vi "AudioSetup.vi"() -> ()   [LabVIEW 2014]
uses:
  Element.ctl
  States.ctl
  <vilib>/Analysis/4window.llb/windowTd.ctl
  <vilib>/Instr/_visa.llb/VISA Configure Serial Port (Instr).vi
  <vilib>/Analysis/NI_AALPro.lvlib
  <vilib>/gmath/NI_Gmath.lvlib
panel:
  out "Elements Out":T1[](array[typedef])
  in  "stop":bool
  in  "Offset Volt":dbl
  in  "Visualizers":T2(tab)
  out "Local Signal":dbl[](graph)
  out "Global Signal":dbl[](graph)
  out "Intensity Graph":dbl[][](graph)
  out "Local Signal FFT":dbl[](graph)
  in  "Controls & Indicators":T3(tab)
  in  "Port Config Control":T4={"Baudrate"=2000000, "COM Port"="", "Termination\nCharacter"=10} {"Termination\nCharacter" format="%.0x"}
  in  "ADC Config Control":T5={"Resolution"=8, "VCC"=5.0, "Sampling Frequency"=75000.0, "Data Blocks"=20, "Samples per Block"=200} {"Data Blocks" min=1 max=50000 step=1}
  out "ADC Config Indicator":cluster{"Number of Samples":u32}
  in  "Record Config Control":T6={"index"=76000, "Freq. Res 2"=0.0, "time steps"=-1, "frequency bins"=512, "type"=enum."", "length"=64}
  in  "FFT Config Control":T7={"time steps"=-1, "frequency bins"=512, "length"=64, "Freq. Res"=0.0, "type"=enum."Rectangle"}
  out "count 2":i32
  out "Acquisition Loop":dbl format="%.4p"
  out "VISA Loop":dbl format="%.4p"
  out "FFT Loop":dbl format="%.4p"
  out "Main Loop":dbl format="%.4p"
  in  "Menu Cluster":T8
  in  "Menu Button":bool
  in  "Lock Gate":bool
  in  "Parar":bool
  in  "Gate":bool
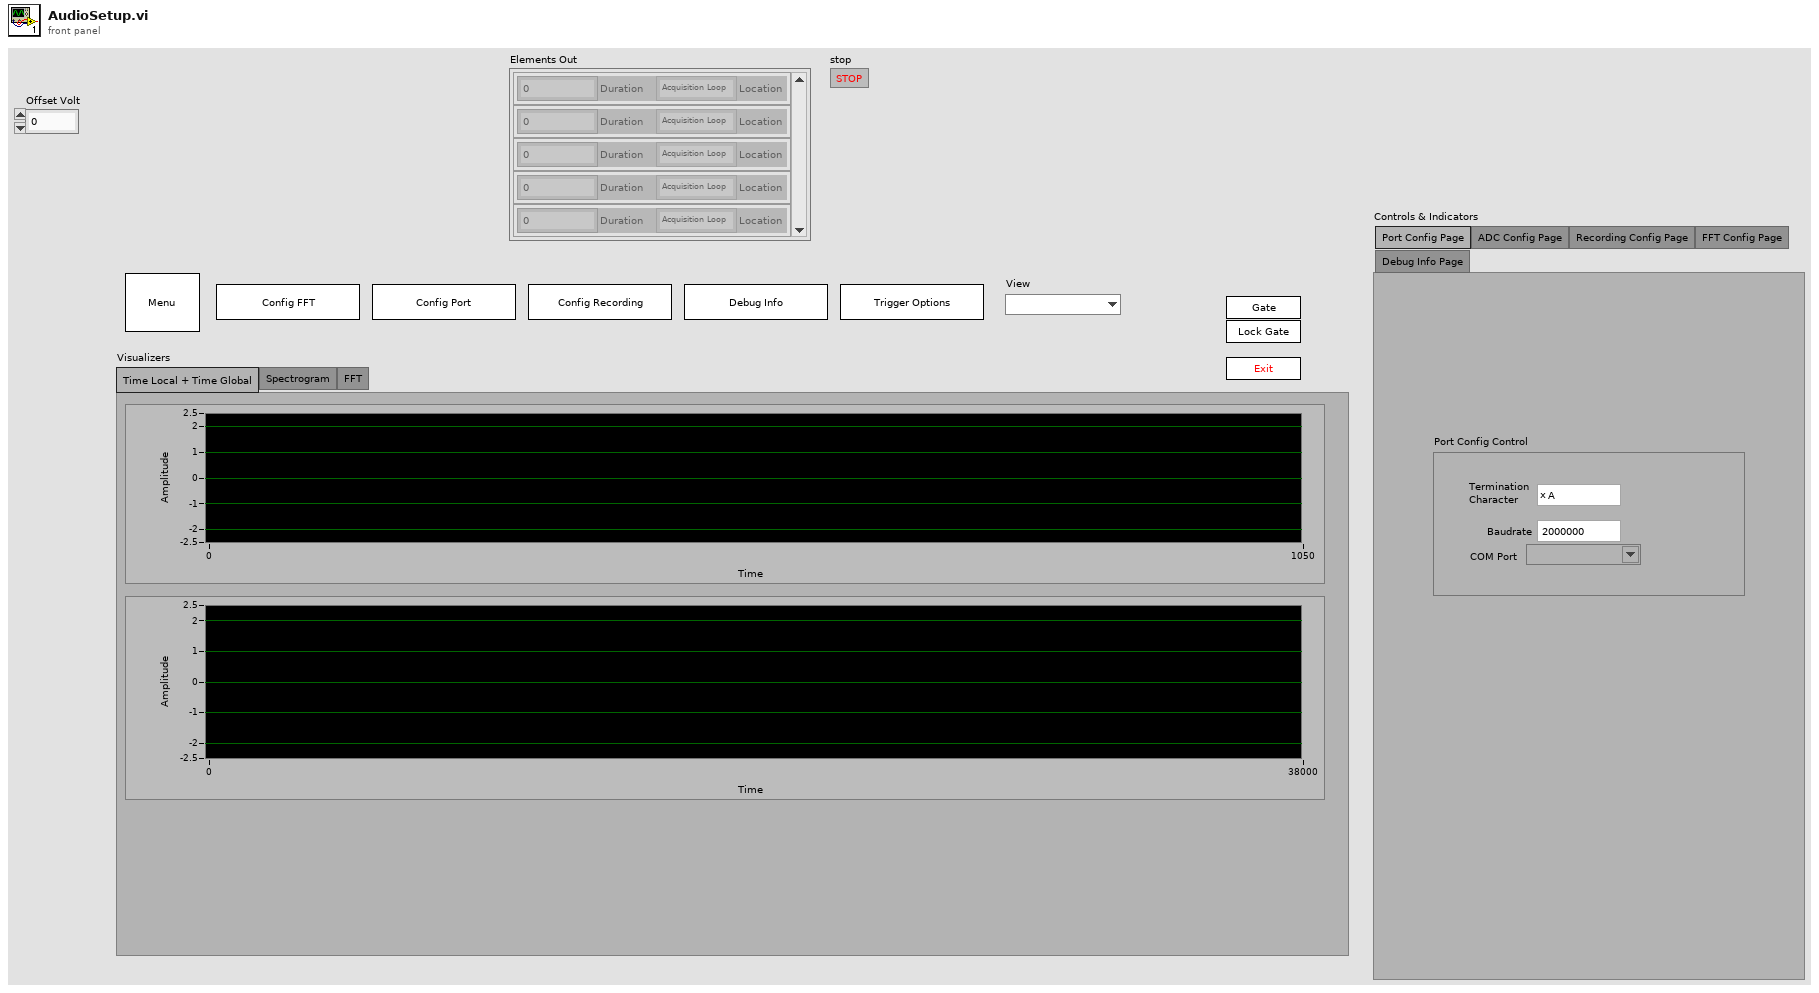
[diagram p1: front panel]
types:
  T1 = typedef "Element.ctl" = cluster{"Duration":dbl, "Location":enum16{"Acquisition Loop", "VISA Loop", "FFT Loop", "Spectrogram Loop"}}
  T2 = enum32{"Time Local + Time Global", "Spectrogram", "FFT"}
  T3 = enum32{"Port Config Page", "ADC Config Page", "Recording Config Page", "FFT Config Page", "Debug Info Page"}
  T4 = cluster{"Baudrate":u32, "COM Port":refnum<visa-resource-name>, "Termination\nCharacter":u8}
  T5 = cluster{"Resolution":i16, "VCC":dbl, "Sampling Frequency":dbl, "Data Blocks":u32, "Samples per Block":u32}
  T6 = cluster{"index":i32, "Freq. Res 2":dbl, "time steps":i32, "frequency bins":i32, "type":enum16{""}, "length":i32}
  T7 = cluster{"time steps":i32, "frequency bins":i32, "length":i32, "Freq. Res":dbl, "type":enum16{"Rectangle", "Hanning", "Hamming", "Blackman-Harris", "Exact Blackman", "Blackman", "Flat Top", "4 Term B-Harris ", "7 Term B-Harris", "Low Sidelobe", "Blackman Nuttall", "Triangle", "Bartlett-Hanning", "Bohman", "Parzen", "Welch", "Kaiser", "Dolph-Chebyshev", "Gaussian"}}
  T8 = cluster{"Configure FFT Parameters":bool, "Configure Comunication Port":bool, "Recording Options":bool, "Debug Info":bool, "Trigger Options":bool, "View":enum16{""}}
  T9 = typedef "States.ctl" = enum16{"Init", "Flush", "Add"}
  T10 = typedef "NI_AALPro.lvlib/windowTd.ctl" = enum16{"Rectangle", "Hanning", "Hamming", "Blackman-Harris", "Exact Blackman", "Blackman", "Flat Top", "4 Term B-Harris ", "7 Term B-Harris", "Low Sidelobe", "Blackman Nuttall", "Triangle", "Bartlett-Hanning", "Bohman", "Parzen", "Welch", "Kaiser", "Dolph-Chebyshev", "Gaussian"}
  T11 = enum16{"Rectangle", "Hanning", "Hamming", "Blackman-Harris", "Exact Blackman", "Blackman", "Flat Top", "4 Term B-Harris ", "7 Term B-Harris", "Low Sidelobe", "Blackman Nuttall", "Triangle", "Bartlett-Hanning", "Bohman", "Parzen", "Welch", "Kaiser", "Dolph-Chebyshev", "Gaussian"}
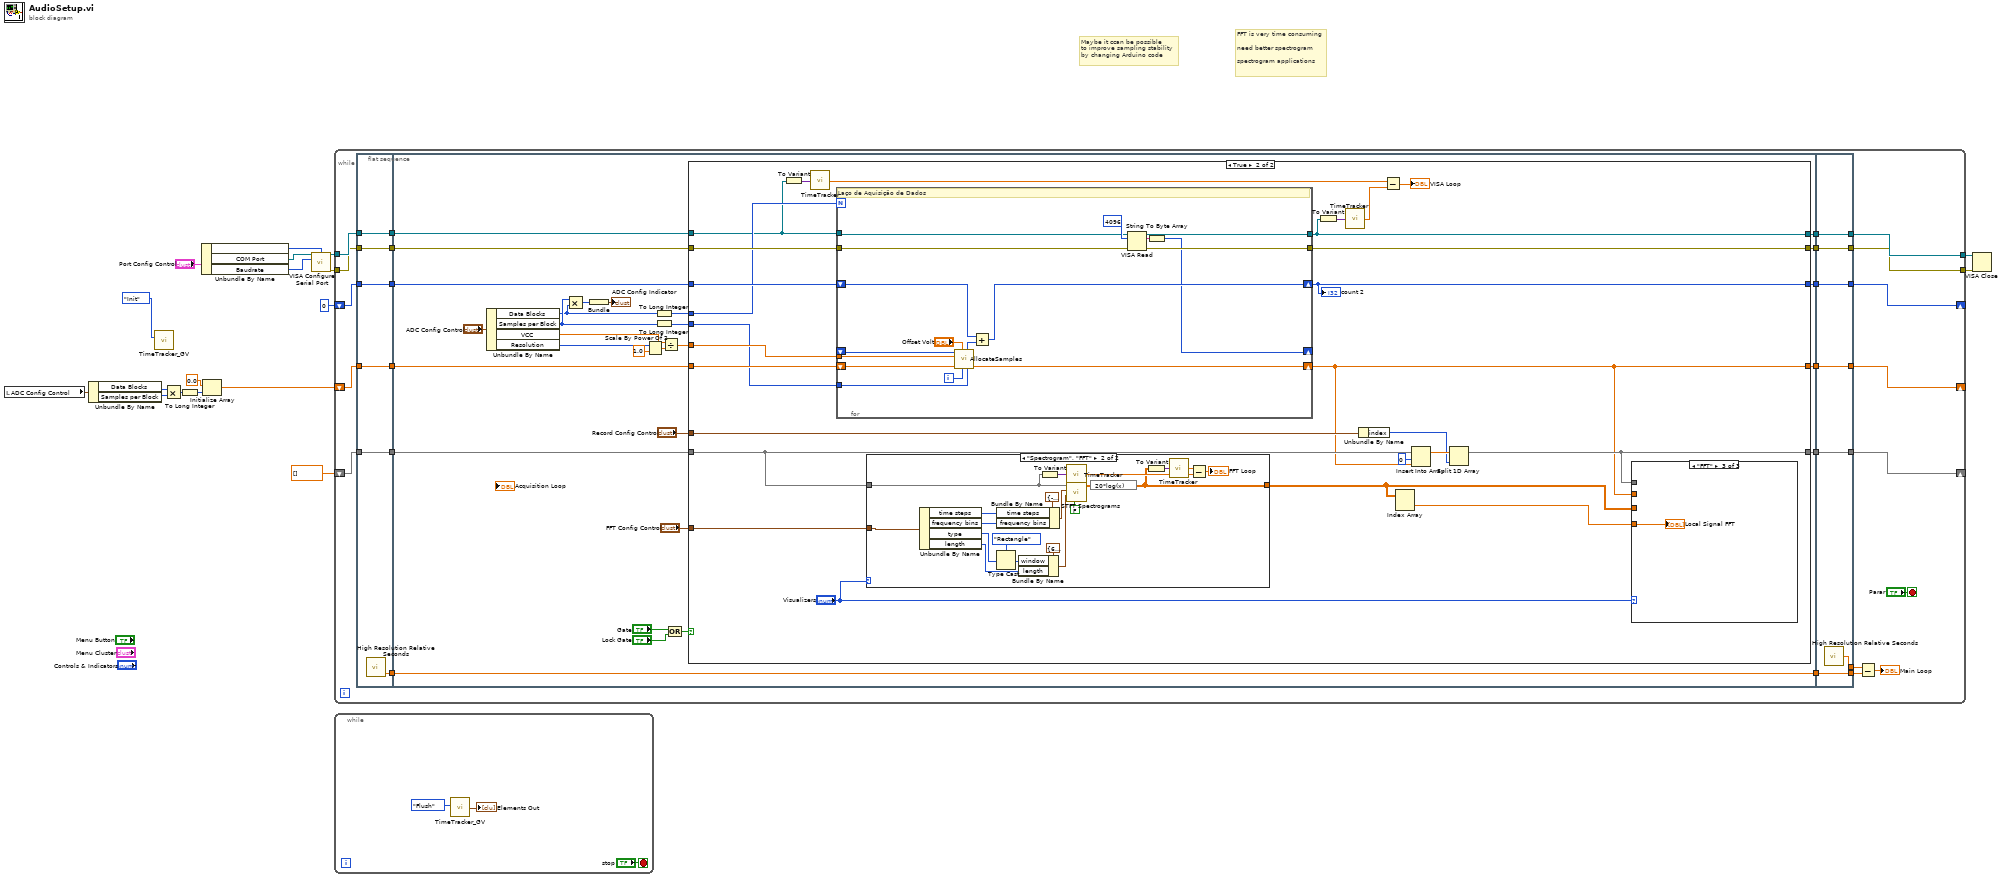
[diagram p0: block diagram]
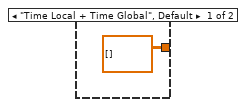
[diagram p3: hidden frame]
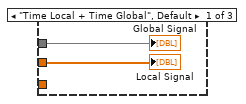
[diagram p4: hidden frame]
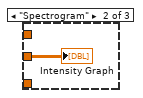
[diagram p5: hidden frame]
diagram:
  # "FFT is very time consuming\n\nneed better spectrogram\n\nspectrogram applications"
  # "Maybe it ccan be possible \nto improve sampling stability \nby changing Arduino code"
  n1 = local read "ADC Config Control"() -> (w5:T5)
  n2 = Unbundle By Name(w5) -> ("Data Blocks"=w4:u32, "Samples per Block"=w3:u32)
  n3 = call "TimeTracker_GV.vi"("Action"=States."Init") -> ()  [unwired: 6 in, 1 out]
  n4 = Multiply(x=w4, y=w3) -> (x*y=w2:u32)
  n5 = To Long Integer(number=w2) -> (32bit integer=w12:i32)
  n6 = Unbundle By Name("Port Config Control") -> ("Termination\nCharacter"=w8:u8, "COM Port"=w7:refnum<visa-resource-name>, "Baudrate"=w6:u32)
  n7 = Initialize Array(0.0 ("dimension size"), w12) -> (w13:dbl[])
  n8 = call-poly "VISA Configure Serial Port"("VISA resource name"=w7, "termination char\n(0xA = '\\n' = LF)"=w8, "baud rate (9600)"=w6) -> ("VISA resource name out"=w18:refnum<visa-resource-name>, "error out"=w17:errorcluster)  [unwired: 11 in]
  n9 = while {
    tunnel: w18 -> [w44]
    tunnel: w17 -> [w41]
    tunnel: [w43] -> w16
    tunnel: [w42] -> w15
    shift-right: [w38] -> _
    shift-left: 0 ("dimension size") -> [w39]
    shift-right: [w37] -> _
    shift-left: w13 -> [w40]
    shift-right: [w36] -> _
    shift-left: dbl[] [] -> [w35]
    stop <- "Parar" stop-if-true
    n10 = flat-sequence {
      tunnel: w35 -> [w46]
      tunnel: w39 -> [w47]
      tunnel: w40 -> [w48]
      tunnel: w41 -> [w49]
      tunnel: w44 -> [w50]
      tunnel: [w50] -> w29
      tunnel: [w49] -> w28
      tunnel: [w48] -> w27
      tunnel: [w47] -> w26
      tunnel: [w46] -> w25
      tunnel: [w45] -> w21
      tunnel: [w77] -> w34
      tunnel: [w76] -> w33
      tunnel: [w69] -> w32
      tunnel: [w68] -> w31
      tunnel: [w67] -> w30
      tunnel: w29 -> [w78]
      tunnel: w28 -> [w72]
      tunnel: w27 -> [w71]
      tunnel: w26 -> [w70]
      tunnel: w25 -> [w66]
      tunnel: w21 -> [w51]
      tunnel: [w51] -> w20
      tunnel: [w154] -> w36
      tunnel: [w155] -> w37
      tunnel: [w156] -> w38
      tunnel: [w157] -> w42
      tunnel: [w158] -> w43
      tunnel: w34 -> [w158]
      tunnel: w33 -> [w157]
      tunnel: w32 -> [w156]
      tunnel: w31 -> [w155]
      tunnel: w30 -> [w154]
      tunnel: [w153] -> w22
      tunnel: w20 -> [w152]
      tunnel: [w152] -> w19
      frame #0 {
        n11 = call <vilib>:"High Resolution Relative Seconds.vi"() -> ("relative seconds"=w45:dbl)
      }
      frame #1 {
        n12 = Unbundle By Name("ADC Config Control") -> ("Data Blocks"=w54:u32, "Samples per Block"=w55:u32, "VCC"=w62:dbl, "Resolution"=w63:i16)
        n13 = Multiply(x=w55, y=w54) -> (x*y=w52:u32)
        n14 = Bundle(w52) -> (→"ADC Config Indicator":cluster{u32})  [unwired: 1 in]
        n15 = Scale By Power Of 2(n=w63, x=1.0) -> (x*2^n=w60:dbl)
        n16 = To Long Integer(number=w54) -> (32bit integer=w56:i32)
        n17 = To Long Integer(number=w55) -> (32bit integer=w57:i32)
        n18 = Divide(x=w62, y=w60) -> (x/y=w59:dbl)
        n19 = Or(x="Gate", y="Lock Gate") -> (x .or. y?=w73:bool)
        n20 = case shown="True" w73 {
          tunnel: w78 -> [w83 w87]
          tunnel: w72 -> [w82 w108]
          tunnel: [w83 w88] -> w77
          tunnel: [w82 w109] -> w76
          tunnel: w71 -> [w80 w107]
          tunnel: w70 -> [w81 w106]
          tunnel: [w81 w105] -> w69
          tunnel: w59 -> [_ w104]
          tunnel: [w80 w99] -> w68
          tunnel: [w79 w102] -> w67
          tunnel: w66 -> [w79 w103]
          tunnel: "FFT Config Control" -> [_ w101]
          tunnel: "Record Config Control" -> [_ w100]
          tunnel: w57 -> [_ w98]
          tunnel: w56 -> [_ w97]
          frame False {
          }
          frame True {
            n21 = To Variant(anything=w87) -> (Variant=w89:variant)
            n22 = call "TimeTracker.vi"("Ref In"=w89) -> ("Time Out"=w86:dbl)  [unwired: 4 in]
            n23 = for {
              N: w97 -> [_]
              tunnel: w87 -> [w140]
              tunnel: w108 -> [w146]
              tunnel: [w141] -> w88
              tunnel: [w145] -> w109
              shift-right: [w132] -> w99
              shift-left: w107 -> [w131]
              tunnel: w98 -> [w133]
              shift-right: [w143] -> w105
              shift-left: w106 -> [w142]
              shift-right: [w139] -> _
              shift-left: _ -> [w137]
              tunnel: w104 -> [w136]
              i -> [w135]
              # "Laço de Aquisição de Dados"
              n24 = call "AllocateSamples.vi"("Samples per Block"=w133, "Loop Iteration"=w135, "Offset Volt"="Offset Volt", "Converted Array In"=w131, "Conversion Constant"=w136, "Raw Array In"=w137) -> ("Converted Array out"=w132:dbl[], "Missed Samples"=w134:i32)  [unwired: 3 in, 1 out]
              n25 = Add(x=w142, y=w134) -> (x+y=w143:i32)
              n26 = VISA Read(VISA resource name=w140, byte count=u32 4096, error in (no error)=w146) -> (VISA resource name out=w141:refnum<visa-resource-name>, read buffer=w144:string, error out=w145:errorcluster)  [unwired: 1 out]
              n27 = String To Byte Array(string=w144) -> (unsigned byte array=w139:u8[])
            }
            "count 2" <- w105
            n28 = case shown="\"Spectrogram\", \"FFT\"" "Visualizers" {
              tunnel: w101 -> [_ w117]
              tunnel: [dbl[][] [] ("STFT Spectrogram {X}") w113] -> w96
              tunnel: w103 -> [_ w111]
              frame "Time Local + Time Global", Default {
              }
              frame "Spectrogram", "FFT" {
                n29 = Unbundle By Name(w117) -> ("time steps"=w126:i32, "frequency bins"=w125:i32, "type"=w119:T11, "length"=w123:i32)
                n30 = Type Cast(type=windowTd."Rectangle", x=w119) -> (*(type *) &x=w120:T10)
                n31 = Bundle By Name(cluster=cluster{"time steps":i32, "frequency bins":i32} {"time steps"=-1, "frequency bins"=512} ("time-freq sampling info"), "time steps"=w126, "frequency bins"=w125) -> (w124:cluster{"time steps":i32, "frequency bins":i32})
                n32 = Bundle By Name(cluster=cluster{"length":i32, "window":T10} {"length"=64, "window"=enum."Rectangle"} ("window info"), "window"=w120, "length"=w123) -> (w122:cluster{"length":i32, "window":T10})
                n33 = To Variant(anything=w111) -> (Variant=w112:variant)
                n34 = call "TimeTracker.vi"("Ref In"=w112) -> ("Time Out"=w115:dbl)  [unwired: 4 in]
                n35 = call <vilib>:"STFT Spectrograms.vi"("energy conservation?"=FALSE, "window info"=w122, "time-freq sampling info"=w124, "X"=w111) -> ("STFT Spectrogram {X}"=w128:dbl[][])  [unwired: 6 in, 1 out]
                n36 = expression code="20*log(x)"(w128) -> (w113:dbl[][])
                n37 = To Variant(anything=w113) -> (Variant=w114:variant)
                n38 = call "TimeTracker.vi"("Ref In"=w114) -> ("Time Out"=w116:dbl)  [unwired: 4 in]
                n39 = Subtract(x=w116, y=w115) -> (x-y=→"FFT Loop":dbl)
              }
            }
            n40 = To Variant(anything=w88) -> (Variant=w90:variant)
            n41 = call "TimeTracker.vi"("Ref In"=w90) -> ("Time Out"=w85:dbl)  [unwired: 4 in]
            n42 = Unbundle By Name(w100) -> ("index"=w91:i32)
            n43 = Subtract(x=w86, y=w85) -> (x-y=→"VISA Loop":dbl)
            n44 = Index Array(array=w96) -> (element=w95:dbl[])  [unwired: 2 in]
            n45 = Insert Into Array(array=w103, index=0, new element=w99) -> (w92:dbl[])
            n46 = Split 1D Array(array=w92, index=w91) -> (first subarray=w102:dbl[])  [unwired: 1 out]
            n47 = case shown="\"FFT\"" "Visualizers" {
              tunnel: w99 -> [w148 _ _]
              tunnel: w102 -> [w149 _ _]
              tunnel: w96 -> [_ w150 _]
              tunnel: w95 -> [_ _ w151]
              frame "Time Local + Time Global", Default {
                "Local Signal" <- w148
                "Global Signal" <- w149
              }
              frame "Spectrogram" {
                "Intensity Graph" <- w150
              }
              frame "FFT" {
                "Local Signal FFT" <- w151
              }
            }
          }
        }
      }
      frame #2 {
        n48 = call <vilib>:"High Resolution Relative Seconds.vi"() -> ("relative seconds"=w153:dbl)
      }
    }
    n49 = Subtract(x=w22, y=w19) -> (x-y=→"Main Loop":dbl)
  }
  n50 = while {
    stop <- "stop" stop-if-true
    n51 = call "TimeTracker_GV.vi"("Action"=States."Flush") -> ("Elements Out"=→"Elements Out":T1[])  [unwired: 6 in]
  }
  n52 = VISA Close(VISA resource name=w16, error in (no error)=w15) -> ()  [unwired: 1 out]
